vi "Actor Core.vi"(8 "error in":errorcluster, 11 "Instrument Actor in":refnum<class "Instrument Actor.lvclass">) -> (0 "error out":errorcluster, 3 "Actor out":refnum<class "Actor.lvclass">)   [LabVIEW 2016, in "Instrument Actor.lvclass"]
doc: "(<B>Filename</B>: Actor Framework.lvlib:Actor.lvclass:Actor Core.vi)\n\nReceives messages to the actor, reacts to them, and initiates any error handling that may shut the actor down.\n\nDescendant classes may override this VI to append parallel tasks for the actor to complete while it handles messages. Overrides use the Call Parent Method node."
uses:
  Instrument Actor.lvclass
  C:/Program Files (x86)/National Instruments/LabVIEW 2016/vi.lib/ActorFramework/Actor/Actor.lvclass
  G:/sw_repo/For Builds/Reusable/SuperActor/SuperActor.lvclass
  <vilib>/ActorFramework/Actor/Actor.lvclass
  <vilib>/ActorFramework/Actor/Actor.lvclass/Actor.ctl
  Instrument Actor.lvclass/Instrument Actor.ctl
  SuperActor/SuperActor.lvclass/SuperActor.ctl
  Instrument.lvclass/Instrument.ctl
  Generic Update Data MSG/Generic Update Data MSG.lvclass/Generic Update Data MSG.ctl
  <vilib>/ActorFramework/Message Enqueuer/Message Enqueuer.lvclass/Message Enqueuer.ctl
  Generic Update Data MSG/Write ID.vi
  Generic Update Data MSG/Write Data.vi
  Read Instr.vi
  SuperActor/Read CVT Session.vi
  Read Update Data.vi
  SuperActor/Read ID.vi
  Read ExtCom.vi
  Read Data Notifier.vi
  Generic Update Data MSG/Generic Update Data MSG.lvclass
  C:/Program Files (x86)/National Instruments/LabVIEW 2016/vi.lib/ActorFramework/Message/Message.lvclass
  <vilib>/ActorFramework/Message Priority Queue/Priority Enqueue.vi
  SuperActor/SuperActor.lvclass
  Instrument.lvclass
  Session APIs/_Session Fwk/Session - Root.lvclass
  Data/Data.lvclass
  Session APIs/CVT/CVT.lvclass
  <vilib>/ActorFramework/Message Enqueuer/Message Enqueuer.lvclass
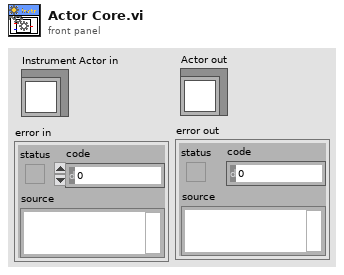
[diagram p1: front panel]
types:
  T1 = typedef "Session - Root.lvclass/Session Handle.ctl" = refnum<data-value>
  T2 = cluster{"tag":string, "section":string, "data":variant}
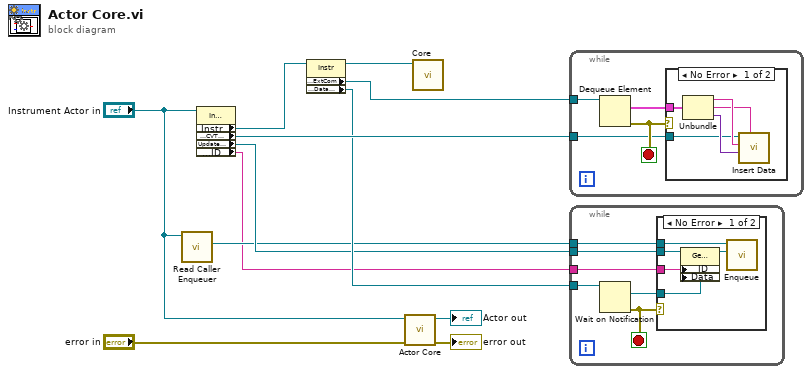
[diagram p0: block diagram]
diagram:
  n1 = call <vilib>:"Read Caller Enqueuer.vi"("Actor"="Instrument Actor in") -> ("Caller Enqueuer"=w2:refnum<class "Message Enqueuer.lvclass">)  [unwired: 10 in]
  n2 = property class="Instrument Actor"(reference="Instrument Actor in") -> ("Instr"=w7:refnum<class "Instrument.lvclass">, "Accessors:CVT Session"=w6:T1, "Update Data"=w4:refnum<class "Generic Update Data MSG.lvclass">, "Accessors:ID"=w1:string)  [unwired: 1 in, 2 out]
  n3 = property class="Instr"(reference=w7) -> (reference out=w9:refnum<class "Instrument.lvclass">, "Accessors:ExtCom"=w8:refnum<queue>, "Accessors:Data Notifier"=w5:refnum<notifier>)  [unwired: 1 in, 1 out]
  n4 = call-parent "Actor Core.vi"("error in"="error in", "Actor in"="Instrument Actor in") -> ("error out"=→"error out":errorcluster, "Actor out"=→"Actor out":refnum<class "Actor.lvclass">)  [unwired: 8 in]
  n5 = call "Core.vi"("Instr in"=w9) -> ()  [unwired: 11 in]
  n6 = while {
    tunnel: w8 -> [w16]
    tunnel: w6 -> [w13]
    stop <- w14 stop-if-true
    n7 = Dequeue Element(queue=w16) -> (element=w15:T2, error out=w14:errorcluster)  [unwired: 2 in, 2 out]
    n8 = case shown="No Error" w14 {
      tunnel: w15 -> [w21 _]
      tunnel: w13 -> [w17 _]
      frame No Error {
        n9 = Unbundle(w21) -> ("tag"=w20:string, "section"=w19:string, "data"=w18:variant)
        n10 = call "Insert Data.vi"("Group"=w19, "Data"=w18, "tag"=w20, "CVT Session In"=w17) -> ()  [unwired: 6 in, 2 out]
      }
      frame Error {
      }
    }
  }
  n11 = while {
    tunnel: w5 -> [w27]
    tunnel: w4 -> [w25]
    tunnel: w2 -> [w23]
    tunnel: w1 -> [w22]
    stop <- w26 stop-if-true
    n12 = Wait on Notification(notifier=w27) -> (notification=w24:refnum<class "Data.lvclass">, error out=w26:errorcluster)  [unwired: 3 in, 2 out]
    n13 = case shown="No Error" w26 {
      tunnel: w25 -> [w32 _]
      tunnel: w24 -> [w28 _]
      tunnel: w23 -> [w30 _]
      tunnel: w22 -> [w29 _]
      frame No Error {
        n14 = property class="Generic Update Data MSG"(reference=w32, "ID"=w29, "Data"=w28) -> (reference out=w31:refnum<class "Generic Update Data MSG.lvclass">)  [unwired: 1 in, 1 out]
        n15 = call <vilib>:"Enqueue.vi"("Message"=w31, "Message Enqueuer in"=w30) -> ()  [unwired: 8 in, 2 out]
      }
      frame Error {
      }
    }
  }
